vi "On The Fly analysis.vi"() -> ()   [LabVIEW 2020]
uses:
  Instance           7 27Saved   On The Fly analysis .vi
  Instance           1 27Saved   On The Fly analysis .vi
panel:
  out "Simulated Waveform Frequency":dynamicdata(graph)
  out "error out":errorcluster
  in  "stop":bool
  out "Waveform Chart":dynamicdata(graph)
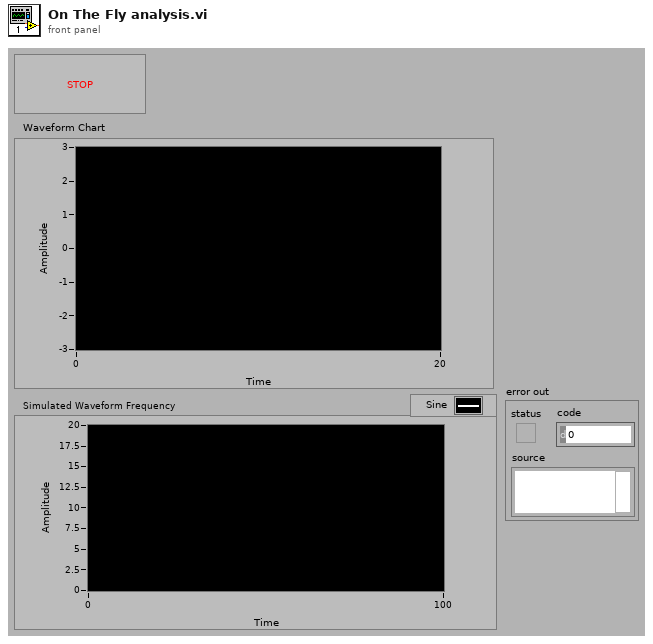
[diagram p1: front panel]
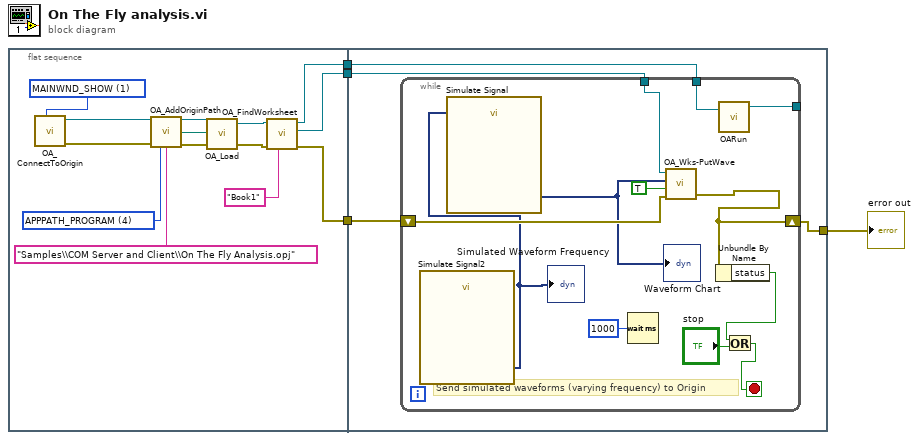
[diagram p0: block diagram]
diagram:
  n1 = flat-sequence {
    tunnel: [w14] -> w4
    tunnel: [w10] -> w3
    tunnel: [w8] -> w2
    tunnel: w4 -> [w20]
    tunnel: w3 -> [w22]
    tunnel: w2 -> [w21]
    tunnel: [w19] -> w1
    frame #0 {
      w7 = 1 items=["MAINWND_HIDE"=0, "MAINWND_SHOW"=1, "MAINWND_SHOWMINIMIZED"=2, "MAINWND_SHOWMAXIMIZED"=3, "MAINWND_SHOW_BRING_TO_FRONT"=100] ("Visible")
      w18 = 4 items=["APPPATH_USER"=2, "APPPATH_GROUP"=3, "APPPATH_PROGRAM"=4] ("Type")
      n2 = call "OA_ConnectToOrigin.vi"("Visible"=w7) -> ("error out"=w5:errorcluster, "Origin.IOApplication"=w6:refnum<k7>)  [unwired: 7 in]
      n3 = call "OA_AddOriginPath.vi"("Origin.IOApplication"=w6, "error in (no error)"=w5, "Type"=w18, "Filename"="Samples\\COM Server and Client\\On The Fly Analysis.opj") -> ("Origin.IOApplication"=w17:refnum<k7>, "path out"=w16:path, "error out"=w12:errorcluster)  [unwired: 9 in]
      n4 = call "OA_Load.vi"("error in (no error)"=w12, "Path"=w16, "Origin.IOApplication"=w17) -> ("error out"=w9:errorcluster, "Origin.IOApplication"=w11:refnum<k7>)  [unwired: 1 out]
      n5 = call "OA_FindWorksheet.vi"("Name"="Book1", "error in (no error)"=w9, "Origin.IOApplication"=w11) -> ("error out"=w8:errorcluster, "Origin.Worksheet"=w10:refnum<k7>, "Origin.IOApplication"=w14:refnum<k7>)  [unwired: 6 in]
    }
    frame #1 {
      n6 = while {
        shift-right: [w23] -> w19
        shift-left: w21 -> [w33]
        tunnel: w22 -> [w28]
        tunnel: w20 -> [w26]
        tunnel: [w25] -> _
        stop <- w31 stop-if-true
        # "Send simulated waveforms (varying frequency) to Origin"
        n7 = call "Simulate Signal2"() -> ("Sine"=w24:dynamicdata)  [unwired: 14 in, 1 out]
        "Simulated Waveform Frequency" <- w24
        n8 = call "Simulate Signal"("Frequency"=w24) -> ("Sine with Uniform Noise"=w29:dynamicdata)  [unwired: 13 in, 1 out]
        "Waveform Chart" <- w29
        n9 = Wait (ms)(milliseconds to wait=u32 1000) -> ()  [unwired: 1 out]
        n10 = call "OA_Wks-PutWave.vi"("Origin.Worksheet"=w28, "Dynamic Data"=w29, "Append to existing data in column"=TRUE, "error in (no error)"=w33) -> ("error IO"=w23:errorcluster)  [unwired: 2 in, 1 out]
        n11 = Unbundle By Name(w23) -> ("status"=w30:bool)
        n12 = call "OARun.vi"("Origin.IOApplication"=w26) -> ("Origin.IOApplication"=w25:refnum<k7>)  [unwired: 1 in, 2 out]
        n13 = Or(x=w30, y="stop") -> (x .or. y?=w31:bool)
      }
    }
  }
  "error out" <- w1
